vi "Add cluster section.vi"(8 "error in (no error)":errorcluster, 9 "Name (none)":string, 10 "Array Positions (none)":i32[](array[numeric]), 11 "Data in":T2 {"Device Ref" format="%.0x"; "Section Ref" format="%.0x"}) -> (0 "error out":errorcluster, 1 "Section Ptr":T1=18446744073709551615 format="%.0x", 2 "Item name":string, 3 "Data out":T2 {"Device Ref" format="%.0x"; "Section Ref" format="%.0x"})   [LabVIEW 2016, in "DCM System Explorer.lvlib"]
uses:
  DCM System Explorer.lvlib
  <vilib>/NI Veristand/Custom Device API/Custom Device Item Ref.ctl
  <vilib>/NI VeriStand/Custom Device API/Custom Device API.lvlib
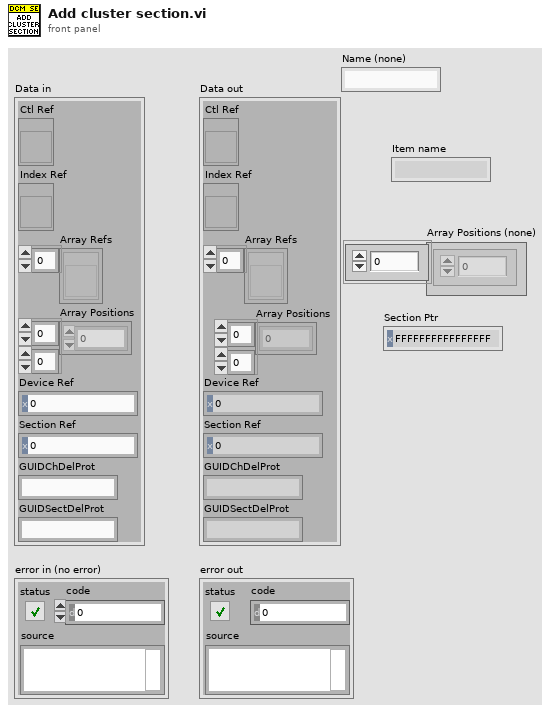
[diagram p1: front panel]
types:
  T1 = typedef "Custom Device API.lvlib/Custom Device Item Ref.ctl" = u64
  T2 = cluster{"Ctl Ref":refnum<vi>, "Index Ref":refnum<vi>, "Array Refs":refnum<vi>[], "Array Positions":i32[][], "Device Ref":T1, "Section Ref":T1, "GUIDChDelProt":string, "GUIDSectDelProt":string}
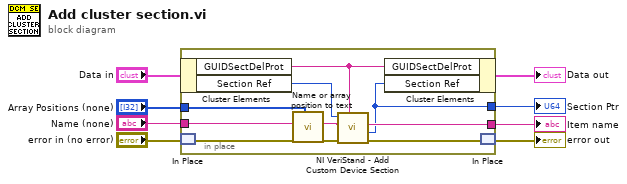
[diagram p0: block diagram]
diagram:
  n1 = in-place {
    in-place-border: "Array Positions (none)" -> [w12]
    in-place-border: [w11] -> w3
    in-place-border: [w10] -> w2
    in-place-border: "Name (none)" -> [w9]
    n2 = in-place-cluster #1("Data in") -> ("GUIDSectDelProt"=w15:string, "Section Ref"=w16:T1)
    n3 = in-place-match #2("error in (no error)") -> (w14:errorcluster)
    n4 = call "Name or array position to text.vi"("Array Positions (none)"=w12, "Name in"=w9) -> ("Name out"=w11:string)  [unwired: 9 in]
    n5 = call <vilib>:"NI VeriStand - Add Custom Device Section.vi"("GUID (Default Section)"=w15, "error in (no error)"=w14, "Section Name"=w11, "Parent Ref in"=w16) -> ("error out"=w13:errorcluster, "Section Ptr"=w10:T1)  [unwired: 4 in, 2 out]
    n6 = in-place-cluster #1("GUIDSectDelProt"=w15, "Section Ref"=w10) -> (→"Data out":T2)
    n7 = in-place-match #2(w13) -> (→"error out":errorcluster)
  }
  "Item name" <- w3
  "Section Ptr" <- w2
